vi "Open In Memory.vi"(8 "error in (no error)":errorcluster, 9 "Mode":T1, 11 "Database Manager in":refnum<class "Database Manager.lvclass">) -> (0 "error out":errorcluster, 3 "Database Manager out":refnum<class "Database Manager.lvclass">)   [LabVIEW 2019, in "HierDAL Library.lvlib" / "Database.lvlib" / "Database Manager.lvclass"]
doc: "Opens in-memory database and initialises it.\n \n<b>Mode</b> - The mode of operation (e.g., Create, Replace, Open, ReadOnly).\n <b>Create</b> - Creates a new database. If the database file already exists, it will be overwritten.\n <b>Replace</b> - Replaces the existing database with a new one.\n <b>Open</b> - Opens an existing database without modifying it.\n <b>Read Only</b> - Opens the database in read-only mode."
uses:
  Database Manager.lvclass
  Controls/Mode.ctl
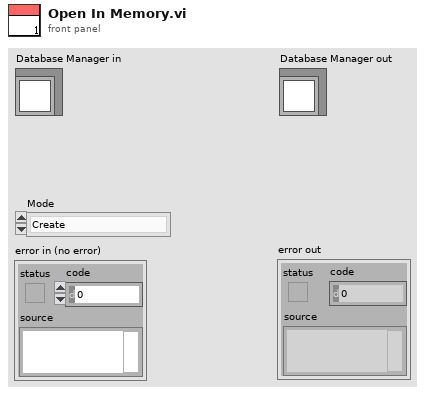
[diagram p1: front panel]
types:
  T1 = typedef "HierDAL Library.lvlib/Database.lvlib/Database Manager.lvclass/Mode.ctl" = enum16{"Create", "Replace", "Open", "Read Only"}
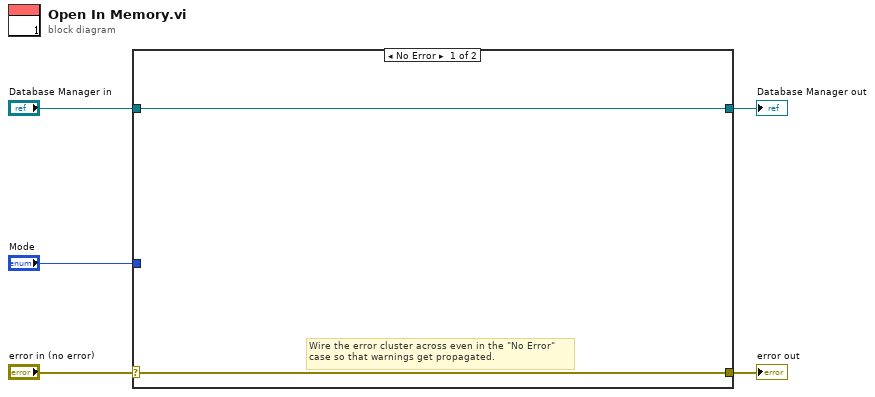
[diagram p0: block diagram]
diagram:
  n1 = case shown="No Error" "error in (no error)" {
    selector: "error in (no error)" -> [w6 w9]
    tunnel: [w6 w9] -> w5
    tunnel: [w7 w8] -> w2
    tunnel: "Database Manager in" -> [w7 w8]
    tunnel: "Mode" -> [_ _]
    frame No Error {
      # "Wire the error cluster across even in the \"No Error\"\ncase so that warnings get propagated."
    }
    frame Error {
    }
  }
  "error out" <- w5
  "Database Manager out" <- w2
